vi "DAQmx.Dark.Current.SubVI.SendData.vi"(0 "Write Pin Task In":refnum<k21>, 1 "Data Pin Task In":refnum<k21>, 2 "Sync Pin Task In":refnum<k21>, 3 "Clear Pin Task In":refnum<k21>, 5 "Data to Send in":u32[](array[numeric])=[1, 2, 4, 8, 16, 32, 64, 128]) -> (6 "Write Pin Task Out":refnum<k21>, 7 "Data Pin Task Out":refnum<k21>, 8 "Sync Pin Task Out":refnum<k21>)   [LabVIEW 2020]
uses:
  <vilib>/DAQmx/write.llb/DAQmx Write (Digital Bool 1Line 1Point).vi
  <vilib>/DAQmx/write.llb/DAQmx Write (Digital U32 1Chan 1Samp).vi
  <vilib>/DAQmx/miscellaneous.llb/DAQmx Fill In Error Info.vi
panel:
  out "Clear Pin Task Out":refnum<k21>
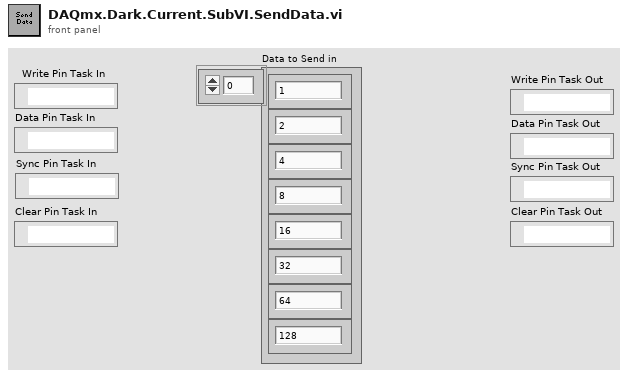
[diagram p1: front panel]
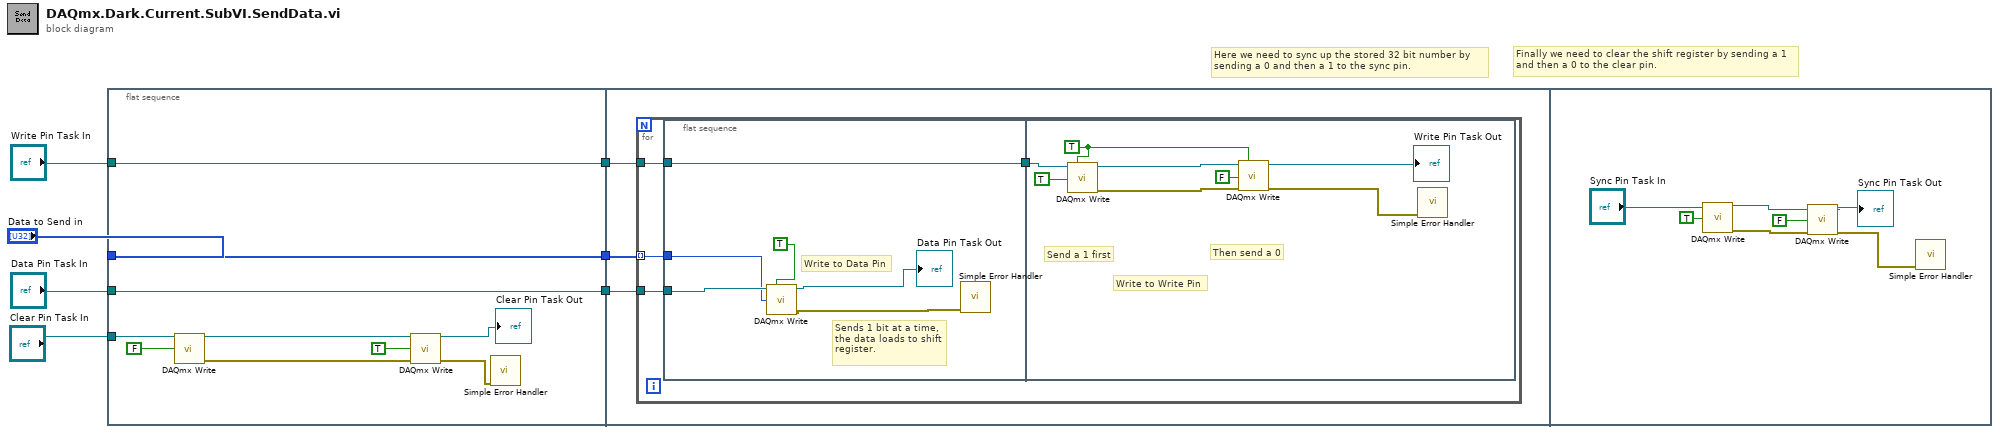
[diagram p0: block diagram]
diagram:
  # "Finally we need to clear the shift register by sending a 1\nand then a 0 to the clear pin."
  # "Here we need to sync up the stored 32 bit number by \nsending a 0 and then a 1 to the sync pin."
  n1 = flat-sequence {
    tunnel: "Data to Send in" -> [w15]
    tunnel: "Data Pin Task In" -> [w16]
    tunnel: "Write Pin Task In" -> [w17]
    tunnel: [w17] -> w4
    tunnel: [w16] -> w3
    tunnel: [w15] -> w2
    tunnel: "Clear Pin Task In" -> [w8]
    tunnel: w4 -> [w20]
    tunnel: w3 -> [w19]
    tunnel: w2 -> [w18]
    frame #0 {
      n2 = call-poly <vilib>:"DAQmx Write.vi"("task/channels in"=w8, "data"=FALSE) -> ("task out"=w12:refnum<k21>, "error out"=w11:errorcluster)  [unwired: 11 in, 1 out]
      n3 = call-poly <vilib>:"DAQmx Write.vi"("task/channels in"=w12, "data"=TRUE, "error in"=w11) -> ("task out"=→"Clear Pin Task Out":refnum<k21>, "error out"=w9:errorcluster)  [unwired: 10 in, 1 out]
      n4 = call <vilib>:"Simple Error Handler.vi"("error in (no error)"=w9) -> ()  [unwired: 4 in, 5 out]
    }
    frame #1 {
      n5 = for {
        tunnel: w20 -> [w24]
        tunnel: w19 -> [w22]
        tunnel: w18 -> [w21] mode=indexing
        n6 = flat-sequence {
          tunnel: w24 -> [w30]
          tunnel: [w30] -> w23
          tunnel: w22 -> [w29]
          tunnel: w21 -> [w28]
          tunnel: w23 -> [w36]
          frame #0 {
            # "Sends 1 bit at a time,\nthe data loads to shift\nregister."
            # "Write to Data Pin"
            n7 = call-poly <vilib>:"DAQmx Write.vi"("task/channels in"=w29, "auto start"=TRUE, "data"=w28) -> ("task out"=→"Data Pin Task Out":refnum<k21>, "error out"=w25:errorcluster)  [unwired: 10 in, 1 out]
            n8 = call <vilib>:"Simple Error Handler.vi"("error in (no error)"=w25) -> ()  [unwired: 4 in, 5 out]
          }
          frame #1 {
            w31 = TRUE
            # "Then send a 0"
            # "Send a 1 first"
            # "Write to Write Pin"
            n9 = call-poly <vilib>:"DAQmx Write.vi"("task/channels in"=w36, "auto start"=w31, "data"=TRUE) -> ("task out"=w32:refnum<k21>, "error out"=w33:errorcluster)  [unwired: 10 in, 1 out]
            n10 = call-poly <vilib>:"DAQmx Write.vi"("task/channels in"=w32, "auto start"=w31, "data"=FALSE, "error in"=w33) -> ("task out"=→"Write Pin Task Out":refnum<k21>, "error out"=w34:errorcluster)  [unwired: 9 in, 1 out]
            n11 = call <vilib>:"Simple Error Handler.vi"("error in (no error)"=w34) -> ()  [unwired: 4 in, 5 out]
          }
        }
      }
    }
    frame #2 {
      n12 = call-poly <vilib>:"DAQmx Write.vi"("task/channels in"="Sync Pin Task In", "data"=TRUE) -> ("task out"=w39:refnum<k21>, "error out"=w40:errorcluster)  [unwired: 11 in, 1 out]
      n13 = call-poly <vilib>:"DAQmx Write.vi"("task/channels in"=w39, "data"=FALSE, "error in"=w40) -> ("task out"=→"Sync Pin Task Out":refnum<k21>, "error out"=w41:errorcluster)  [unwired: 10 in, 1 out]
      n14 = call <vilib>:"Simple Error Handler.vi"("error in (no error)"=w41) -> ()  [unwired: 4 in, 5 out]
    }
  }
